vi "ShowHideScrollBar.vi"(8 "error in":errorcluster, 11 "reference":refnum<vi>) -> (0 "error out":errorcluster, 1 "Visible?":bool, 2 "Value":string, 3 "reference out":refnum<vi>)   [LabVIEW 2013]
doc: "This VI compares the number of displayed items in the list with the total number of visible rows and shows/hides the Vertical Scroll Bar as appropriate."
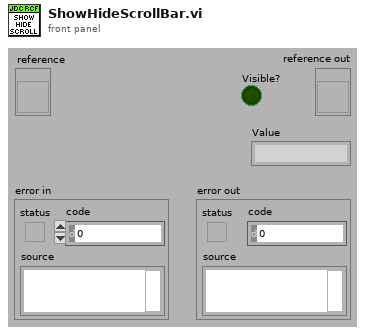
[diagram p1: front panel]
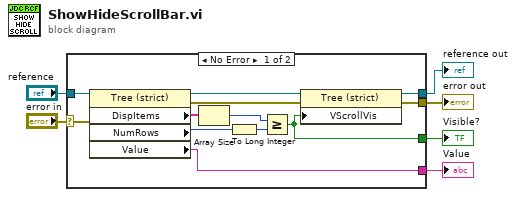
[diagram p0: block diagram]
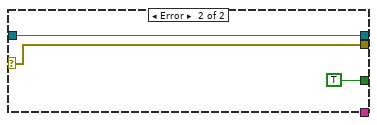
[diagram p2: hidden frame]
diagram:
  n1 = case shown="No Error" "error in" {
    selector: "error in" -> [w8 w21]
    tunnel: "reference" -> [w12 w20]
    tunnel: [w11 _] -> w5
    tunnel: [w10 w20] -> w4
    tunnel: [w9 w21] -> w2
    tunnel: [w7 TRUE] -> w1
    frame No Error {
      n2 = property class="Tree (strict)"(reference=w12, error in=w8) -> (reference out=w16:refnum<vi>, error out=w15:errorcluster, "DispItems"=w14:string[], "NumRows"=w18:u32, "Value"=w11:string)
      n3 = Array Size(array=w14) -> (size(s)=w17:i32)
      n4 = To Long Integer(number=w18) -> (32bit integer=w13:i32)
      n5 = Greater Or Equal?(x=w17, y=w13) -> (x >= y?=w7:bool)
      n6 = property class="Tree (strict)"(reference=w16, error in=w15, "VScrollVis"=w7) -> (reference out=w10:refnum<vi>, error out=w9:errorcluster)
    }
    frame Error {
    }
  }
  "Value" <- w5
  "reference out" <- w4
  "error out" <- w2
  "Visible?" <- w1
